vi "Robot Global Data.vi"() -> ()   [LabVIEW 2018]
doc: "This global VI can contain as many global variables as you need. Place a control on the panel, give it a good name. To read or write to it from a VI, drag the icon to the diagram of that VI. You can also drag from the project. Click on the node to change which global you access. You shouldn't have multiple locations writing to a global or it will cause a race-condition."
uses:
  <vilib>/Rock Robotics/WPI/Camera/WPI_CameraImageSize.ctl
  <vilib>/Rock Robotics/WPI/DriverStation/WPI_DriverStationRobotMode2.ctl
  LabVIEW_is_Under_Control.lib/Util/Unpack Gamepad/Button Cluster.ctl
  LabVIEW_is_Under_Control.lib/Util/Unpack Gamepad/Axes Cluster.ctl
  LabVIEW_is_Under_Control.lib/Util/Unpack Gamepad/D-Pad.ctl
panel:
  in  "Auto Rotate":bool
  in  "Right Auto":dbl
  in  "Left Auto":dbl
  in  "Yaw 2":dbl
  in  "Auto Forward":bool
  in  "Yaw":dbl
  in  "Encoder direita":dbl
  in  "Reset Yaw and Encoders":bool
  in  "Wheel Auto":dbl
  in  "Throttle Auto":dbl
  in  "Reset Climber Encoder":bool
  in  "Back Speed":dbl
  in  "Front Speed":dbl
  in  "Climber Encoder":dbl
  in  "Climber Limit":bool
  in  "Elevador Height":dbl
  in  "Elevador Limit":bool
  in  "Intake Pos":dbl
  in  "Setpoint Elevador":dbl
  in  "Cargo In?":bool
  in  "Intake limit":bool
  in  "Hatch In?":bool
  out "D-Pad":T1
  in  "Intake Speed":dbl
  in  "Empurrador":bool
  in  "Espatula":bool
  in  "Climber Pivot":bool
  in  "Setpoint Intake":dbl
  out "Axes - Joy 1":T2
  out "Axes - Joy 0":T2
  out "Buttons - Joy 0":T3
  out "Buttons - Joy 1":T3
  in  "Robot Mode":T4
  in  "image size":T5=enum."320x240"
  in  "Enable Vision":bool
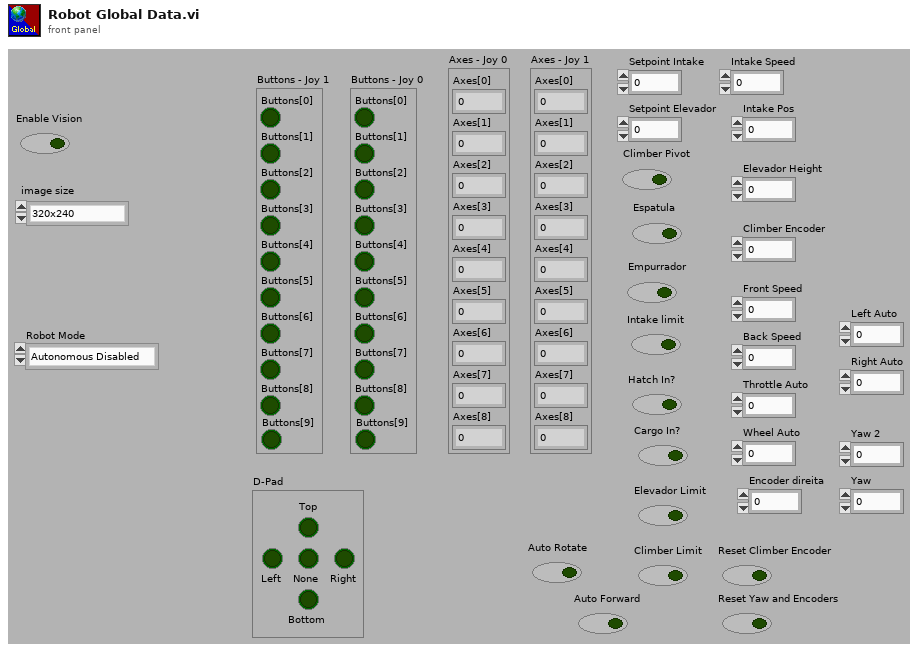
[diagram p1: front panel]
types:
  T1 = typedef "D-Pad.ctl" = cluster{"Top":bool, "Bottom":bool, "None":bool, "Right":bool, "Left":bool}
  T2 = typedef "Axes Cluster.ctl" = cluster{"Axes[0]":dbl, "Axes[1]":dbl, "Axes[2]":dbl, "Axes[3]":dbl, "Axes[4]":dbl, "Axes[5]":dbl, "Axes[6]":dbl, "Axes[7]":dbl, "Axes[8]":dbl}
  T3 = typedef "Button Cluster.ctl" = cluster{"Buttons[0]":bool, "Buttons[1]":bool, "Buttons[2]":bool, "Buttons[3]":bool, "Buttons[4]":bool, "Buttons[5]":bool, "Buttons[6]":bool, "Buttons[7]":bool, "Buttons[8]":bool, "Buttons[9]":bool}
  T4 = typedef "WPI_DriverStationRobotMode2.ctl" = enum16{"Autonomous Disabled", "Autonomous Enabled", "Teleop Disabled", "Teleop Enabled", "Disconnected", "Finish", "Test Disabled", "Test Enabled", "Emergency Stopped"}
  T5 = typedef "WPI_CameraImageSize.ctl" = enum16{"640x480", "320x240", "160x120", "Custom"}
diagram:
